vi "IMU RT Driver VI.vi"() -> ()   [LabVIEW 2015, in "IMU Custom Device.lvlib"]
uses:
  IMU Custom Device.lvlib
  <vilib>/NI Veristand/Custom Device API/Custom Device Item Ref.ctl
  <vilib>/NI Veristand/Custom Device API/Custom Device Channel Type.ctl
  <vilib>/NI Veristand/Custom Device API/Message Response (String).ctl
  <vilib>/NI Veristand/Custom Device API/Message Response (Byte Array).ctl
  <vilib>/NI Veristand/Custom Device API/Custom Device API.lvlib
  <vilib>/NI Veristand/Custom Device Tools/Custom Device Utility Library/Custom Device Utility Library.lvlib
panel:
  in  "Initialization Status Notifier":refnum<notifier>
  in  "Status Notifier":refnum<notifier>
  in  "Device Outputs FIFO":refnum<k33>
  in  "Device Clock":string
  in  "Device Reference":T1 format="%.0x"
  # "Custom Device Template\nv1.0"
  # "Use this template as a starting point for creating a custom device code module. The input controls shown here are specially named controls that the system will use to provide the device loop with data. The controls are not required for the device loop to run. For instance, if the device doesn't produce any output data, then you don't need the Device Outputs FIFO control. If you do use these controls, however, they need to have these exact names to be functional."
  # "The optional status notifier element is used to notify the RT engine of the last state of the custom device, and to indicate the device has completed execution. If this control is not used, a default No Error value is returned to the system when the device finishes execution.\n\nNote: This error state is not checked until the system shuts down. Use an output status channel to send more immediate status values to the system."
  # "This optional input can be used to send the VeriStand Engine the final status of the custom device initalization process. If this control exists on the custom device front panel, the VeriStand Engine will wait for a status update before starting up. If the custom device reports an error, that will abort the execution of the current configuration in the VeriStand Engine.\n\nThis control can be deleted if the custom device does not need to send the initialization status update."
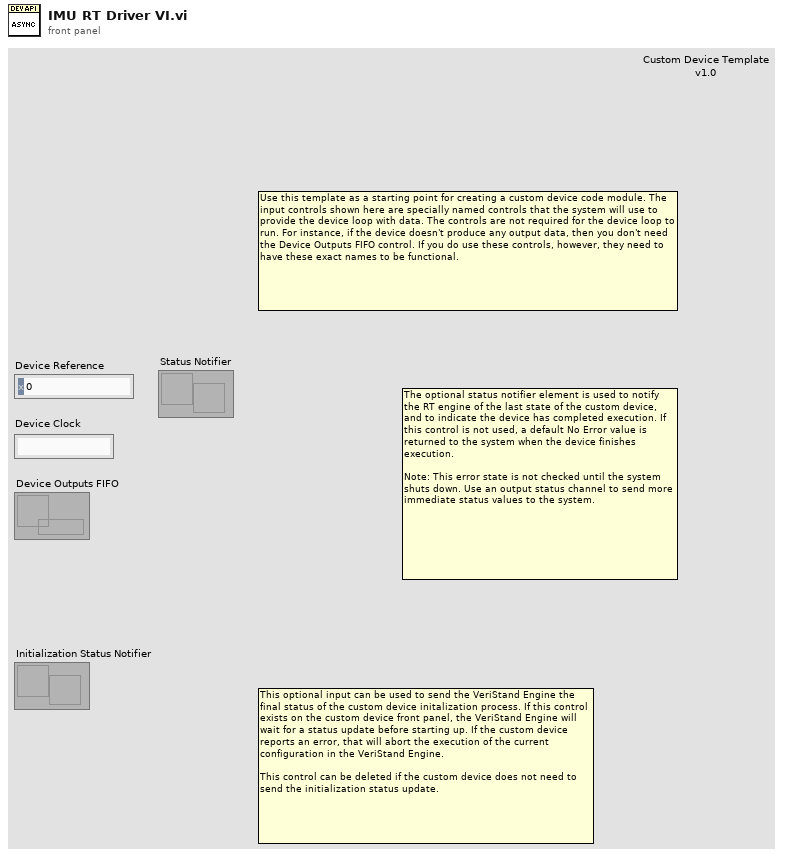
[diagram p1: front panel]
types:
  T1 = typedef "Custom Device API.lvlib/Custom Device Item Ref.ctl" = u64
  T2 = typedef "Custom Device API.lvlib/Custom Device Channel Type.ctl" = enum16{"Input", "Output"}
  T3 = typedef "Custom Device API.lvlib/Custom Device Engine Event Ref.ctl" = refnum<event-registration>
  T4 = typedef "Custom Device API.lvlib/Message Response (String).ctl" = cluster{"Response":string, "Error":errorcluster}
  T5 = typedef "Custom Device API.lvlib/Message Response (Byte Array).ctl" = cluster{"Response":u8[], "Error":errorcluster}
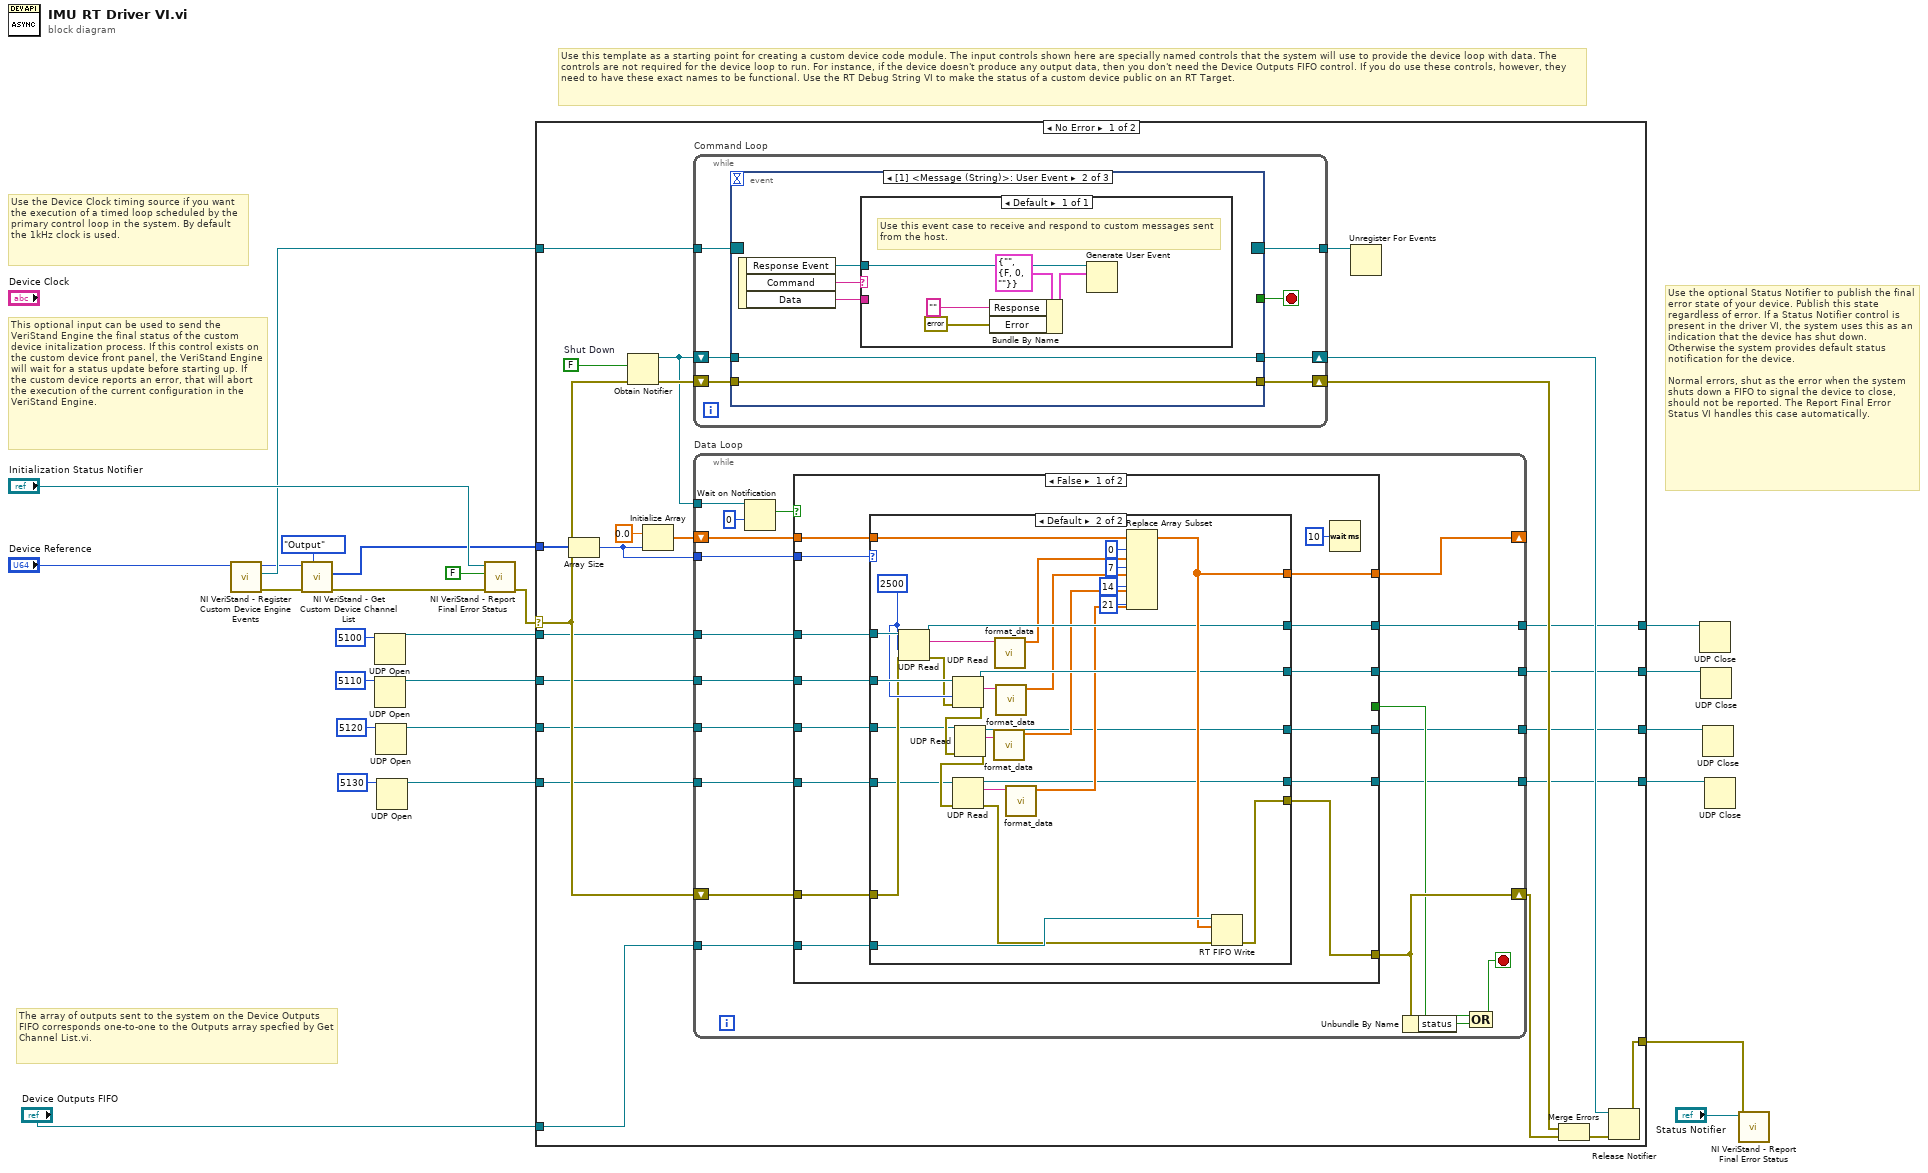
[diagram p0: block diagram]
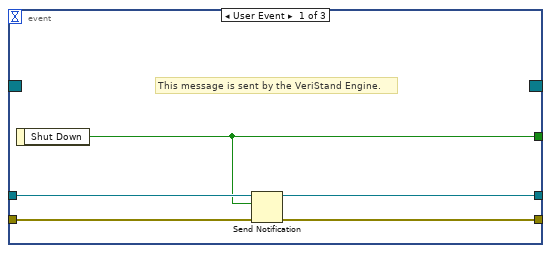
[diagram p2: hidden frame]
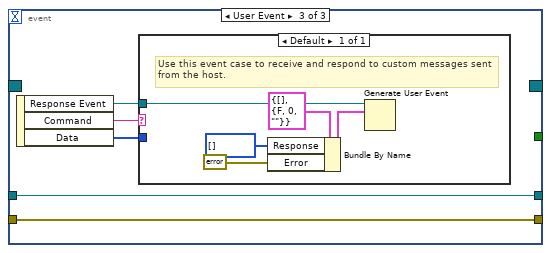
[diagram p3: hidden frame]
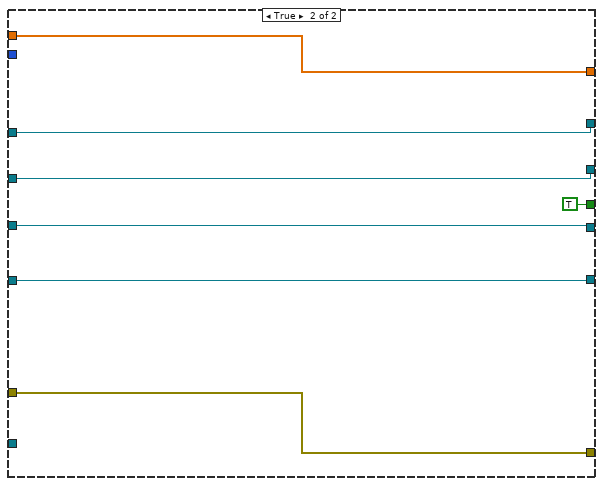
[diagram p5: hidden frame]
diagram:
  # "This optional input can be used to send the VeriStand Engine the final status of the custom device initalization process. If this control exists on the custom device front panel, the VeriStand Engine will wait for a status update before starting up. If the custom device reports an error, that will abort the execution of the current configuration in the VeriStand Engine."
  # "Use the optional Status Notifier to publish the final error state of your device. Publish this state regardless of error. If a Status Notifier control is present in the driver VI, the system uses this as an indication that the device has shut down. Otherwise the system provides default status notification for the device.\n\nNormal errors, shut as the error when the system shuts down a FIFO to signal the device to close, should not be reported. The Report Final Error Status VI handles this case automatically."
  # "The array of outputs sent to the system on the Device Outputs FIFO corresponds one-to-one to the Outputs array specfied by Get Channel List.vi."
  # "Use the Device Clock timing source if you want the execution of a timed loop scheduled by the primary control loop in the system. By default the 1kHz clock is used."
  # "Use this template as a starting point for creating a custom device code module. The input controls shown here are specially named controls that the system will use to provide the device loop with data. The controls are not required for the device loop to run. For instance, if the device doesn't produce any output data, then you don't need the Device Outputs FIFO control. If you do use these controls, however, they need to have these exact names to be functional. Use the RT Debug String VI to make the status of a custom device public on an RT Target."
  n1 = call <vilib>:"NI VeriStand - Register Custom Device Engine Events.vi"("Device Ref in"="Device Reference") -> ("error out"=w25:errorcluster, "Custom Device Engine Event Ref"=w19:T3, "Device Ref out"=w16:T1)  [unwired: 8 in]
  n2 = call <vilib>:"NI VeriStand - Get Custom Device Channel List.vi"("Channel Type"=Custom_Device_Channel_Type."Output", "error in (no error)"=w25, "Device Ref in"=w16) -> ("error out"=w13:errorcluster, "Specified Channel Ref List"=w21:T1[])  [unwired: 7 out]
  n3 = UDP Open(11:u16 5100 ("port")) -> (port=w11:refnum<k16>)  [unwired: 4 in, 2 out]
  n4 = UDP Open(11:u16 5110 ("port")) -> (port=w9:refnum<k16>)  [unwired: 4 in, 2 out]
  n5 = UDP Open(11:u16 5120 ("port")) -> (port=w4:refnum<k16>)  [unwired: 4 in, 2 out]
  n6 = UDP Open(11:u16 5130 ("port")) -> (port=w3:refnum<k16>)  [unwired: 4 in, 2 out]
  n7 = call <vilib>:"NI VeriStand - Report Final Error Status.vi"("error in (no error)"=w13, "Filter FIFO & Shutdown Errors (T)"=FALSE ("Filter FIFO Errors (T)"), "Status Notifier"="Initialization Status Notifier") -> ("error out"=w15:errorcluster)  [unwired: 8 out]
  n8 = case shown="No Error" w15 {
    selector: w15 -> [w37 w164]
    tunnel: "Device Outputs FIFO" -> [w48 _]
    tunnel: w21 -> [w45 _]
    tunnel: w19 -> [w44 _]
    tunnel: [w42 w164] -> w18
    tunnel: w11 -> [w34 w163]
    tunnel: w9 -> [w33 w162]
    tunnel: [w32 w163] -> w8
    tunnel: [w31 w162] -> w7
    tunnel: w4 -> [w29 w161]
    tunnel: w3 -> [w28 w160]
    tunnel: [w27 w161] -> w2
    tunnel: [w26 w160] -> w1
    frame No Error {
      w43 = FALSE  # Shut Down
      n9 = Array Size(array=w45) -> (size(s)=w30:i32)
      n10 = Obtain Notifier(notification data type=w43, error in (no error)=w37) -> (notifier out=w40:refnum<notifier>, error out=w49:errorcluster)  [unwired: 2 in, 1 out]
      n11 = Initialize Array(0.0 ("element"), w30) -> (w46:dbl[])
      n12 = while "Command Loop" {
        tunnel: w44 -> [w56]
        tunnel: [w55] -> w41
        shift-right: [w52] -> w39
        shift-left: w40 -> [w53]
        shift-right: [w50] -> w35
        shift-left: w49 -> [w51]
        stop <- w54 stop-if-true
        n13 = event shown="[1] <Message (String)>: User Event" {
          selector: w56 -> [_ _ _]
          dyn-events: [_ _ _] -> w55
          timeout: _ -> [_ _ _]
          tunnel: [w59 _ _] -> w54
          tunnel: w53 -> [w60 w64 w74]
          tunnel: [w61 w64 w74] -> w52
          tunnel: w51 -> [w58 w62 w72]
          tunnel: [w57 w62 w72] -> w50
          event User Event {
            # "This message is sent by the VeriStand Engine."
            n14 = event-data() -> ("Shut Down"=w59:bool)  [unwired: 1 in]
            n15 = Send Notification(notification=w59, notifier=w60, error in (no error)=w58) -> (notifier out=w61:refnum<notifier>, error out=w57:errorcluster)
          }
          event User Event {
            n16 = event-data() -> ("Response Event"=w63:refnum<user-event>, "Command"=w66:string, "Data"=w65:string)  [unwired: 1 in]
            n17 = case shown="Default" w66 {
              tunnel: w65 -> [_]
              tunnel: w63 -> [w71]
              frame Default {
                # "Use this event case to receive and respond to custom messages sent from the host."
                n18 = Bundle By Name(cluster=T4 {"Response"="", "Error"={"status"=FALSE, "code"=0, "source"=""}} ("event data"), "Response"="", "Error"=errorcluster {"status"=FALSE, "code"=0, "source"=""}) -> (w69:T4)
                n19 = Generate User Event(user event=w71, event data cluster=w69) -> ()  [unwired: 2 in, 2 out]
              }
            }
          }
          event User Event {
            n20 = event-data() -> ("Response Event"=w73:refnum<user-event>, "Command"=w76:string, "Data"=w75:u8[])  [unwired: 1 in]
            n21 = case shown="Default" w76 {
              tunnel: w75 -> [_]
              tunnel: w73 -> [w81]
              frame Default {
                # "Use this event case to receive and respond to custom messages sent from the host."
                n22 = Bundle By Name(cluster=T5 {"Response"=[], "Error"={"status"=FALSE, "code"=0, "source"=""}} ("event data"), "Response"=u8[] [], "Error"=errorcluster {"status"=FALSE, "code"=0, "source"=""}) -> (w78:T5)
                n23 = Generate User Event(user event=w81, event data cluster=w78) -> ()  [unwired: 2 in, 2 out]
              }
            }
          }
        }
      }
      n24 = while "Data Loop" {
        shift-right: [w96] -> w38
        shift-left: w37 -> [w101]
        shift-right: [w99] -> _
        shift-left: w46 -> [w100]
        tunnel: w48 -> [w98]
        tunnel: w40 -> [w95]
        tunnel: w34 -> [w90]
        tunnel: w33 -> [w89]
        tunnel: [w88] -> w32
        tunnel: [w87] -> w31
        tunnel: w30 -> [w86]
        tunnel: w29 -> [w85]
        tunnel: w28 -> [w84]
        tunnel: [w83] -> w27
        tunnel: [w82] -> w26
        stop <- w91 stop-if-true
        n25 = Wait on Notification(notifier=w95, timeout in ms (-1)=0) -> (notification=w94:bool)  [unwired: 2 in, 3 out]
        n26 = case shown="False" w94 {
          tunnel: w101 -> [w111 w159]
          tunnel: w100 -> [w116 w158]
          tunnel: [w115 w158] -> w99
          tunnel: w98 -> [w114 _]
          tunnel: [w113 w159] -> w96
          tunnel: [_ TRUE] -> w92
          tunnel: w90 -> [w110 w156]
          tunnel: w89 -> [w109 w155]
          tunnel: [w108 w156] -> w88
          tunnel: [w107 w155] -> w87
          tunnel: w86 -> [w106 _]
          tunnel: w85 -> [w105 w154]
          tunnel: w84 -> [w104 w153]
          tunnel: [w103 w154] -> w83
          tunnel: [w102 w153] -> w82
          frame False {
            n27 = case shown="Default" w106 {
              tunnel: w114 -> [_ w152]
              tunnel: w116 -> [w122 w149]
              tunnel: [w119 w151] -> w113
              tunnel: [w122 w147] -> w115
              tunnel: w111 -> [w119 w142]
              tunnel: w110 -> [w121 w150]
              tunnel: w109 -> [w120 w148]
              tunnel: [w121 w146] -> w108
              tunnel: [w120 w145] -> w107
              tunnel: w105 -> [w118 w126]
              tunnel: w104 -> [w117 w125]
              tunnel: [w118 w124] -> w103
              tunnel: [w117 w123] -> w102
              frame 0 {
                # "No outputs to write to system. The Device Outputs FIFO is never created in this case, so don't write to it."
              }
              frame Default {
                w144 = 2500 ("timeout ms (25000)")
                n28 = UDP Read(connection ID=w150, timeout ms (25000)=w144, 8:w142) -> (data out=w141:string, error out=w143:errorcluster, 3:w146:refnum<k16>)  [unwired: 1 in, 2 out]
                n29 = UDP Read(connection ID=w148, timeout ms (25000)=w144, 8:w143) -> (data out=w138:string, error out=w135:errorcluster, 3:w145:refnum<k16>)  [unwired: 1 in, 2 out]
                n30 = UDP Read(connection ID=w126, 8:w135) -> (data out=w131:string, error out=w134:errorcluster, 3:w124:refnum<k16>)  [unwired: 2 in, 2 out]
                n31 = UDP Read(connection ID=w125, 8:w134) -> (data out=w132:string, error out=w133:errorcluster, 3:w123:refnum<k16>)  [unwired: 2 in, 2 out]
                n32 = call "format_data.vi"("String"=w131) -> ("Array"=w130:dbl[])  [unwired: 10 in]
                n33 = call "format_data.vi"("String"=w141) -> ("Array"=w140:dbl[])  [unwired: 10 in]
                n34 = call "format_data.vi"("String"=w138) -> ("Array"=w139:dbl[])  [unwired: 10 in]
                n35 = call "format_data.vi"("String"=w132) -> ("Array"=w129:dbl[])  [unwired: 10 in]
                n36 = Replace Array Subset(array=w149, new element #1=w140, index #1=0 ("index"), new element #2=w139, index #2=7 ("index"), new element #3=w130, index #3=14 ("index"), new element #4=w129, index #4=21 ("index")) -> (w147:dbl[])
                n37 = RT FIFO Write(0:w152, 1:w147, 3:w133) -> (11:w151:errorcluster)  [unwired: 1 in, 4 out]
              }
            }
            n38 = Wait (ms)(milliseconds to wait=u32 10) -> ()  [unwired: 1 out]
          }
          frame True {
          }
        }
        n39 = Unbundle By Name(w96) -> ("status"=w93:bool)
        n40 = Compound Arithmetic op=OR(w92, w93) -> (w91:bool)
      }
      n41 = Unregister For Events(event registration refnum=w41) -> ()  [unwired: 1 in, 1 out]
      n42 = Merge Errors(w35, w38) -> (w36:errorcluster)
      n43 = Release Notifier(notifier=w39, error in (no error)=w36) -> (error out=w42:errorcluster)  [unwired: 1 in, 2 out]
    }
    frame Error {
    }
  }
  n44 = UDP Close(connection ID=w8) -> ()  [unwired: 1 in, 2 out]
  n45 = UDP Close(connection ID=w7) -> ()  [unwired: 1 in, 2 out]
  n46 = UDP Close(connection ID=w2) -> ()  [unwired: 1 in, 2 out]
  n47 = UDP Close(connection ID=w1) -> ()  [unwired: 1 in, 2 out]
  n48 = call <vilib>:"NI VeriStand - Report Final Error Status.vi"("error in (no error)"=w18, "Status Notifier"="Status Notifier") -> ()  [unwired: 1 in, 9 out]
